vi "Append Value To Waveform.vi"(8 "dt (ms)":dbl, 9 "Time Stamp":timestamp, 10 "Numeric":dbl, 11 "waveform in":waveform(dbl)) -> (3 "waveform out":waveform(dbl))   [LabVIEW 2018, in "Logger.lvclass"]
uses:
  logger/Logger.lvclass
  <vilib>/Waveform/WDTOps.llb/WDT Number of Waveform Samples DBL.vi
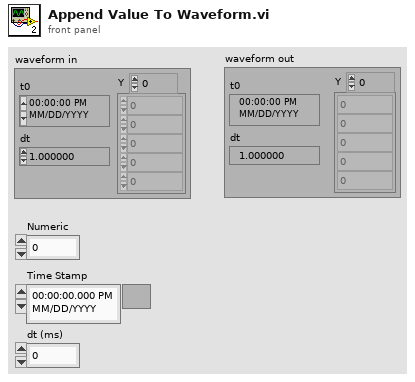
[diagram p1: front panel]
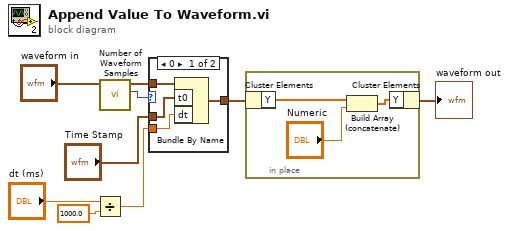
[diagram p0: block diagram]
diagram:
  n1 = Divide(x="dt (ms)", y=1000.0) -> (x/y=w1:dbl)
  n2 = call-poly <vilib>:"Number of Waveform Samples.vi"("waveform in"="waveform in") -> ("number of samples"=w7:i32, "waveform out"=w6:waveform(dbl))  [unwired: 8 in, 1 out]
  n3 = case shown="0" w7 {
    tunnel: w6 -> [w13 w14]
    tunnel: "Time Stamp" -> [w12 _]
    tunnel: [w11 w14] -> w4
    tunnel: w1 -> [w10 _]
    frame 0 {
      n4 = Bundle By Name(cluster=w13, "t0"=w12, "dt"=w10) -> (w11:waveform(dbl))
    }
    frame 1, Default {
    }
  }
  n5 = in-place {
    n6 = in-place-cluster #1(w4) -> ("Y"=w16:dbl[])
    n7 = Build Array (concatenate)(w16, "Numeric") -> (w15:dbl[])
    n8 = in-place-cluster #1("Y"=w15) -> (→"waveform out":waveform(dbl))
  }
